vi "Error Cleanup.vi"(8 "error in (no error)":errorcluster, 11 "Ethernet in":refnum<class "TCP.lvclass">) -> (0 "error out":errorcluster, 3 "Ethernet out":refnum<class "TCP.lvclass">)   [LabVIEW 2018, in "Protocols.lvlib" / "TCP.lvclass"]
uses:
  TCP.lvclass
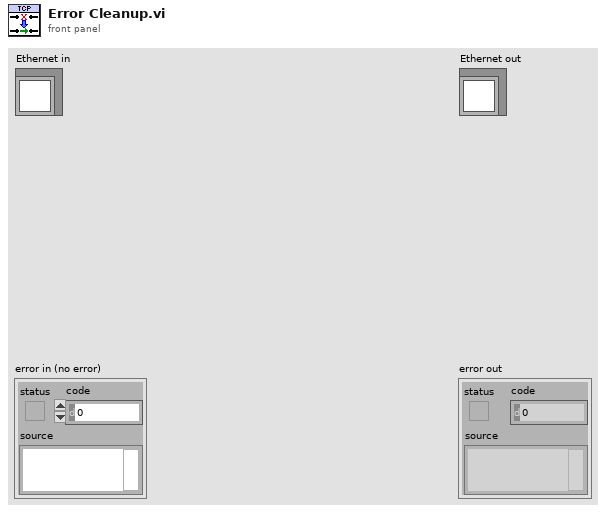
[diagram p1: front panel]
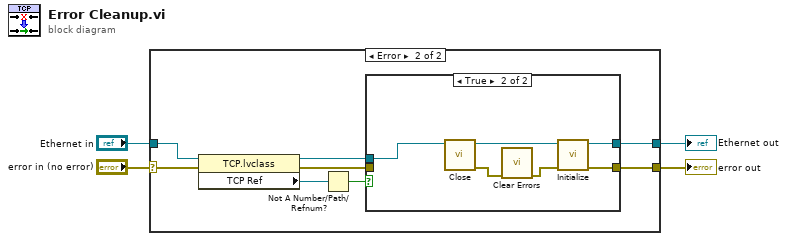
[diagram p0: block diagram]
diagram:
  n1 = case shown="Error" "error in (no error)" {
    selector: "error in (no error)" -> [w6 w13]
    tunnel: "Ethernet in" -> [w5 w14]
    tunnel: [w6 w8] -> w2
    tunnel: [w5 w7] -> w1
    frame No Error {
    }
    frame Error {
      n2 = property class="TCP.lvclass"(reference=w14, error in=w13) -> (reference out=w10:refnum<class "TCP.lvclass">, error out=w9:errorcluster, "TCP Ref"=w12:refnum<k5>)
      n3 = Not A Number/Path/Refnum?(number/path/refnum=w12) -> (NaN/Path/Refnum?=w11:bool)
      n4 = case shown="True" w11 {
        tunnel: w10 -> [w15 w20]
        tunnel: w9 -> [w16 _]
        tunnel: [w16 w22] -> w8
        tunnel: [w15 w21] -> w7
        frame False {
        }
        frame True {
          n5 = call-dynamic "Close.vi"("Ethernet in"=w20) -> ("error out"=w17:errorcluster, "Ethernet out"=w19:refnum<class "TCP.lvclass">)  [unwired: 9 in]
          n6 = call <vilib>:"Clear Errors.vi"("error in (no error)"=w17) -> ("error out"=w18:errorcluster)  [unwired: 5 in, 1 out]
          n7 = call-dynamic "Initialize.vi"("error in (no error)"=w18, "Ethernet in"=w19) -> ("error out"=w22:errorcluster, "Ethernet out"=w21:refnum<class "TCP.lvclass">)  [unwired: 8 in]
        }
      }
    }
  }
  "error out" <- w2
  "Ethernet out" <- w1
